vi "Write Signal Samples to File.vi"() -> ()   [LabVIEW 2014]
uses:
  <vilib>/LabVIEW Universal Transcriptor/LabVIEW to Arduino Transcriptor/Transcriptors/System API/Serial println string.vi
  <vilib>/LabVIEW Universal Transcriptor/LabVIEW to Arduino Transcriptor/Transcriptors/System API/Serial print string.vi
  LabVIEW-Universal-Transcriptor-SD-Card-Library/File.lvclass
  LabVIEW-Universal-Transcriptor-SD-Card-Library/LabVIEW Universal Transcriptor SD Card Library.lvlib
  <vilib>/LabVIEW Universal Transcriptor/LabVIEW for Arduino Math Library/Arduino Math.lvlib
  <vilib>/LabVIEW Universal Transcriptor/LabVIEW to Arduino Transcriptor/Transcriptors/System API/System Serial Library Variables/System Serial Library Variables.lvlib
panel:
  out "gen. signal":u8[](graph)
  out "String Buffer":string
  out "error out":errorcluster
  in  "Error In":errorcluster
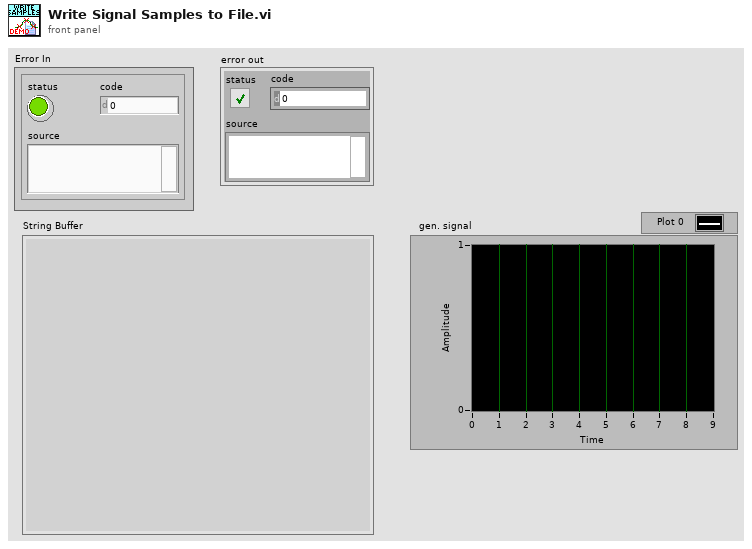
[diagram p1: front panel]
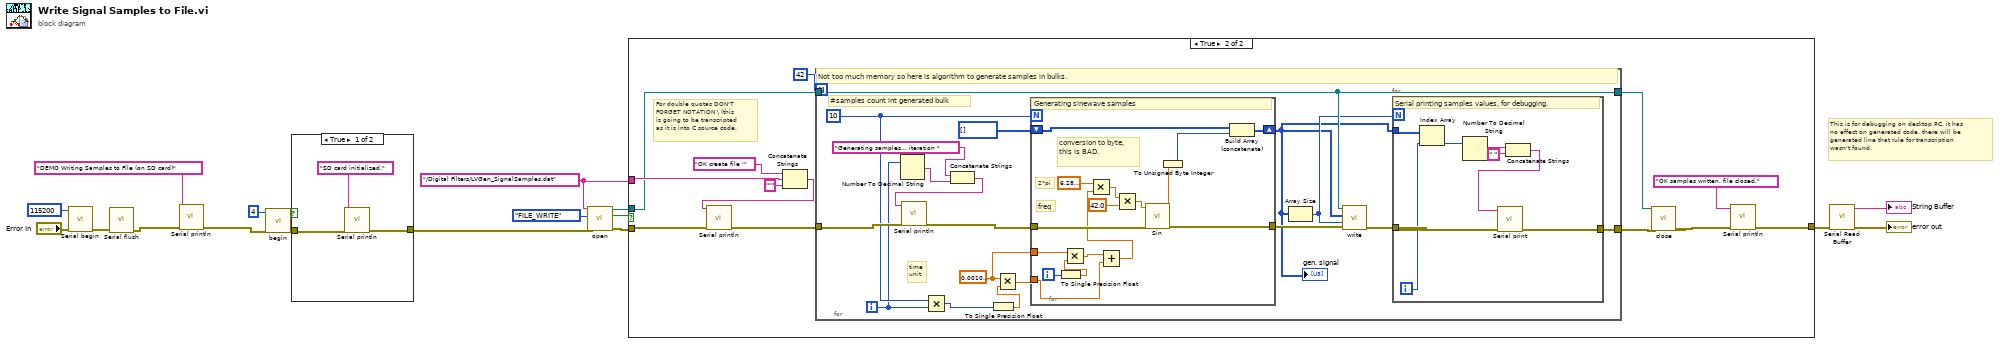
[diagram p0: block diagram]
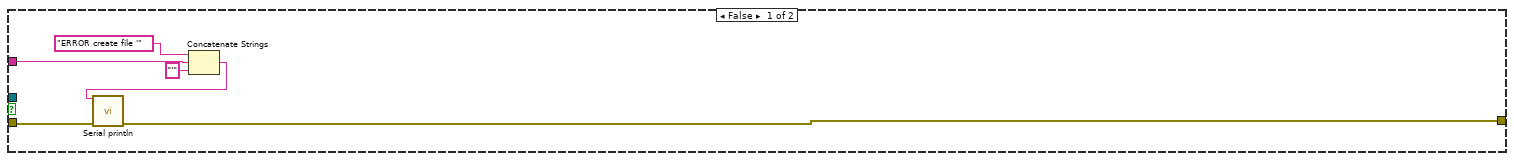
[diagram p2: hidden frame]
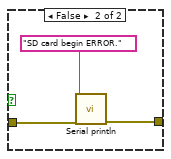
[diagram p3: hidden frame]
diagram:
  w6 = "/Digital Filters/LVGen_SignalSamples.dat" ("filepath")
  # "This is for debugging on desktop PC, it has\nno effect on generated code, there will be\ngenerated line that rule for transcription\nwasn't found."
  n1 = call <vilib>:"Serial begin.vi"("Error In"="Error In", "speed (Bd)"=115200) -> ("Error Out"=w18:errorcluster)  [unwired: 9 in]
  n2 = call <vilib>:"Serial flush.vi"("Error In"=w18) -> ("Error Out"=w16:errorcluster)  [unwired: 10 in]
  n3 = call-poly <vilib>:"Serial println.vi"("Error In"=w16, "string in"="DEMO Writing Samples to File (on SD card)") -> ("Error Out"=w14:errorcluster)  [unwired: 9 in]
  n4 = call <vilib>:"begin.vi"("Error In"=w14, "CS pin (optional)"=u8 4) -> ("Error Out"=w11:errorcluster, "success?"=w12:bool)  [unwired: 8 in]
  n5 = case shown="True" w12 {
    tunnel: w11 -> [w21 w24]
    tunnel: [w19 w22] -> w10
    frame True {
      n6 = call-poly <vilib>:"Serial println.vi"("Error In"=w21, "string in"="SD card initialized.") -> ("Error Out"=w19:errorcluster)  [unwired: 9 in]
    }
    frame False {
      n7 = call-poly <vilib>:"Serial println.vi"("Error In"=w24, "string in"="SD card begin ERROR.") -> ("Error Out"=w22:errorcluster)  [unwired: 9 in]
    }
  }
  n8 = call "open.vi"("Error In"=w10, "mode"=enum16{"FILE_READ", "FILE_WRITE"}."FILE_WRITE", "filepath"=w6) -> ("Error Out"=w8:errorcluster, "opened?"=w7:bool, "File out"=w5:refnum<class "File.lvclass">)  [unwired: 6 in]
  n9 = case shown="True" w7 {
    tunnel: w8 -> [w26 w40]
    tunnel: w6 -> [w30 w39]
    tunnel: [w25 w32] -> w4
    tunnel: w5 -> [_ w37]
    frame False {
      n10 = Concatenate Strings("ERROR create file '" ("string in"), w30, "'" ("string")) -> (w27:string)
      n11 = call-poly <vilib>:"Serial println.vi"("Error In"=w26, "string in"=w27) -> ("Error Out"=w25:errorcluster)  [unwired: 9 in]
    }
    frame True {
      # "For double quotas DON'T\nFORGET NOTATION \\ (this\nis going to be transcripted\nas it is into C source code."
      n12 = Concatenate Strings("OK create file '" ("string in"), w39, "'" ("string")) -> (w41:string)
      n13 = call-poly <vilib>:"Serial println.vi"("Error In"=w40, "string in"=w41) -> ("Error Out"=w38:errorcluster)  [unwired: 9 in]
      n14 = for {
        N: 42 -> [_]
        tunnel: w38 -> [w55]
        tunnel: w37 -> [w56]
        tunnel: [w56] -> w36
        tunnel: [w48] -> w31
        i -> [w45]
        w58 = sgl 0.001 ("x")
        w46 = 10
        # "#samples count int generated bulk"
        # "time\nunit"
        # "Not too much memory so here is algorithm to generate samples in bulks."
        n15 = Number To Decimal String(number=w45) -> (decimal integer string=w53:string)  [unwired: 1 in]
        n16 = Multiply(x=w46, y=w45) -> (x*y=w44:i32)
        n17 = Concatenate Strings("Generating samples... iteration " ("string"), w53) -> (w51:string)
        n18 = call-poly <vilib>:"Serial println.vi"("Error In"=w55, "string in"=w51) -> ("Error Out"=w54:errorcluster)  [unwired: 9 in]
        n19 = To Single Precision Float(number=w44) -> (single precision float=w59:sgl)
        n20 = Multiply(x=w58, y=w59) -> (x*y=w57:sgl)
        n21 = for {
          N: w46 -> [_]
          tunnel: w54 -> [w79]
          shift-right: [w77] -> w47
          shift-left: u8[] [] ("initialized array") -> [w78]
          tunnel: [w76] -> w60
          tunnel: w58 -> [w73]
          tunnel: w57 -> [w72]
          i -> [w85]
          # "conversion to byte, this is BAD."
          # "freq"
          # "2*pi"
          # "Generating sinewave samples"
          n22 = To Single Precision Float(number=w85) -> (single precision float=w81:sgl)
          n23 = Multiply(x=w73, y=w81) -> (x*y=w75:sgl)
          n24 = Add(x=w75, y=w72) -> (x+y=w74:sgl)
          n25 = Multiply(x=sgl 6.28, y=w74) -> (x*y=w83:sgl)
          n26 = Multiply(x=w83, y=sgl 42.0) -> (x*y=w80:sgl)
          n27 = call <vilib>:"Sin.vi"("Error In"=w79, "x"=w80) -> ("Error Out"=w76:errorcluster, "sin(x)"=w71:sgl)  [unwired: 8 in]
          n28 = To Unsigned Byte Integer(number=w71) -> (unsigned 8bit integer=w70:u8)
          n29 = Build Array (concatenate)(w78, w70) -> (w77:u8[])
        }
        "gen. signal" <- w47
        n30 = Array Size(array=w47) -> (size(s)=w49:i32)
        n31 = call-dynamic "write.vi"("error in (no error)"=w60, "length"=w49, "buffer"=w47, "File in"=w56) -> ("error out"=w50:errorcluster)  [unwired: 7 in]
        n32 = for {
          N: w49 -> [_]
          tunnel: w50 -> [w63]
          tunnel: w47 -> [w69]
          tunnel: [w62] -> w48
          i -> [w68]
          # "Serial printing samples values, for debugging."
          n33 = Index Array(array=w69, index=w68) -> (element=w67:u8)
          n34 = Number To Decimal String(number=w67) -> (decimal integer string=w65:string)  [unwired: 1 in]
          n35 = Concatenate Strings(w65, " " ("element")) -> (w64:string)
          n36 = call-poly <vilib>:"Serial print.vi"("Error In"=w63, "string in"=w64) -> ("Error Out"=w62:errorcluster)  [unwired: 9 in]
        }
      }
      n37 = call-dynamic "close.vi"("error in (no error)"=w31, "File in"=w36) -> ("error out"=w33:errorcluster)  [unwired: 9 in]
      n38 = call-poly <vilib>:"Serial println.vi"("Error In"=w33, "string in"="OK samples written, file closed.") -> ("Error Out"=w32:errorcluster)  [unwired: 9 in]
    }
  }
  n39 = call <vilib>:"Serial Read Buffer.vi"("Error In"=w4) -> ("Error Out"=→"error out":errorcluster, "String Buffer"=→"String Buffer":string)  [unwired: 9 in]
